vi "Durchfluss-Druck-Sensoren.vi"(0 "CalGas Ventil":bool, 5 "Istwert Durchfluss":sgl, 7 "Istwert Druck":sgl, 9 "F.Bruch Durchfluss":bool, 11 "F.Bruch Druck":bool, 12 "Analysator aktiv?":bool) -> (4 "Fühlerbruch Durchflusssensor":bool, 6 "Durchfluss":bool, 8 "Fühlerbruch Drucksensor":bool, 10 "Druck CalGas":bool)   [LabVIEW 2020, in "Stoermeldungen.lvlib"]
uses:
  Stoermeldungen.lvlib
  Allgemein/FGV Zustaende Aktionen.ctl
  Funktionstasten/Zustaende.ctl
  Funktionstasten/Funktionstasten.lvlib
  Allgemein/Allgemein.lvlib
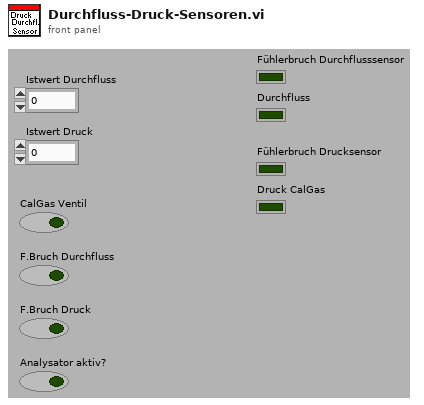
[diagram p1: front panel]
types:
  T1 = typedef "Allgemein.lvlib/FGV Zustaende Aktionen.ctl" = enum16{"lesen", "Zustand PC", "Zustand cRIO", "Bildnummer", "Samplepoint", "Sysloglevel"}
  T2 = typedef "Funktionstasten.lvlib/Zustaende.ctl" = enum16{"Standby", "Pause", "Eco", "Messen", "Kalibrieren", "Spülen Filter", "Spülen Leitung", "Umgebungsluft", "0-Gas", "Cal-Gas", "CG zu PNS", "-------------", "Init 1", "Init 2", "Init 3", "Init 4", "Messen vorbereiten", "Messen durchführen", "Exit"}
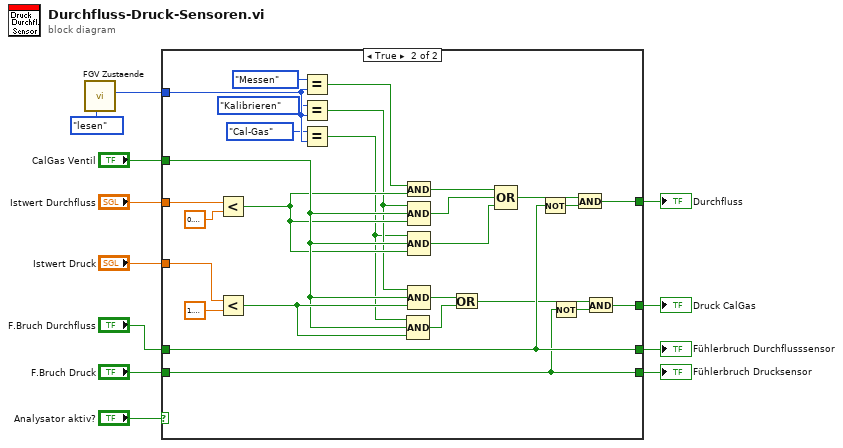
[diagram p0: block diagram]
diagram:
  n1 = call "FGV Zustaende.vi"("Aktionen"=FGV_Zustaende_Aktionen."lesen") -> ("Zustand cRIO"=w1:T2)  [unwired: 6 in, 4 out]
  n2 = case shown="True" "Analysator aktiv?" {
    tunnel: "F.Bruch Durchfluss" -> [_ w24]
    tunnel: [_ w24] -> w6
    tunnel: "Istwert Durchfluss" -> [_ w39]
    tunnel: "CalGas Ventil" -> [_ w31]
    tunnel: [_ w26] -> w3
    tunnel: w1 -> [_ w19]
    tunnel: "Istwert Druck" -> [_ w35]
    tunnel: "F.Bruch Druck" -> [_ w22]
    tunnel: [_ w22] -> w5
    tunnel: [_ w20] -> w4
    frame False {
    }
    frame True {
      n3 = Less?(x=w39, y=sgl 0.3) -> (x < y?=w30:bool)
      n4 = Less?(x=w35, y=sgl 1.3) -> (x < y?=w34:bool)
      n5 = Equal?(x=Zustaende."Messen", y=w19) -> (x = y?=w15:bool)
      n6 = Equal?(x=Zustaende."Kalibrieren", y=w19) -> (x = y?=w14:bool)
      n7 = Equal?(x=Zustaende."Cal-Gas", y=w19) -> (x = y?=w13:bool)
      n8 = And(x=w15, y=w30) -> (x .and. y?=w37:bool)
      n9 = Compound Arithmetic op=AND(w13, w31, w34) -> (w33:bool)
      n10 = Compound Arithmetic op=AND(w14, w31, w30) -> (w29:bool)
      n11 = Compound Arithmetic op=AND(w13, w31, w30) -> (w28:bool)
      n12 = Compound Arithmetic op=AND(w14, w31, w34) -> (w32:bool)
      n13 = Or(x=w32, y=w33) -> (x .or. y?=w21:bool)
      n14 = Compound Arithmetic op=OR(w37, w29, w28) -> (w27:bool)
      n15 = Not(x=w24) -> (.not. x?=w25:bool)
      n16 = Not(x=w22) -> (.not. x?=w23:bool)
      n17 = And(x=w27, y=w25) -> (x .and. y?=w26:bool)
      n18 = And(x=w21, y=w23) -> (x .and. y?=w20:bool)
    }
  }
  "Durchfluss" <- w3
  "Druck CalGas" <- w4
  "Fühlerbruch Drucksensor" <- w5
  "Fühlerbruch Durchflusssensor" <- w6
